vi "Stop_Advise.vi"(0 "error out":errorcluster, 2 "advise refnum":u32) -> ()   [LabVIEW 2012]
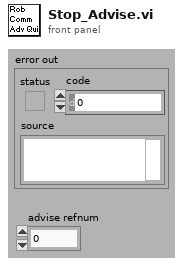
[diagram p1: front panel]
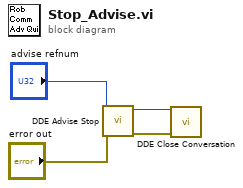
[diagram p0: block diagram]
diagram:
  n1 = call <vilib>:"DDE Advise Stop.vi"("error in (no error)"="error out", "advise refnum"="advise refnum") -> ("error out"=w4:errorcluster, "conversation refnum"=w3:u32)  [unwired: 6 in]
  n2 = call <vilib>:"DDE Close Conversation.vi"("error in (no error)"=w4, "conversation refnum"=w3) -> ()  [unwired: 7 in, 1 out]
